vi "Part 1.vi"(11 "Input":string) -> (3 "Output":i64)   [LabVIEW 2021]
uses:
  d659a181-ebe8-414d-ab0f-685b255bff87.vi
  4776c344-dbbc-458a-98bd-0c10030d5930.vi
  <userlib>/_OpenG.lib/string/string.llb/Convert EOLs (String)__ogtk.vi
  <vilib>/Comparison/Less/Less Functor/Less Functor.lvclass
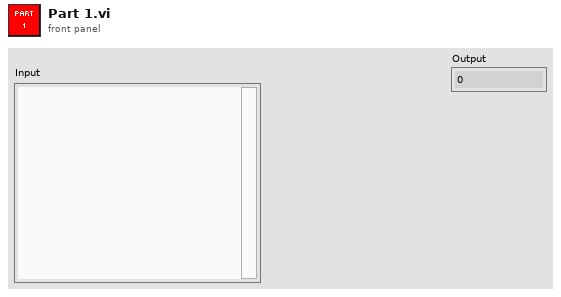
[diagram p1: front panel]
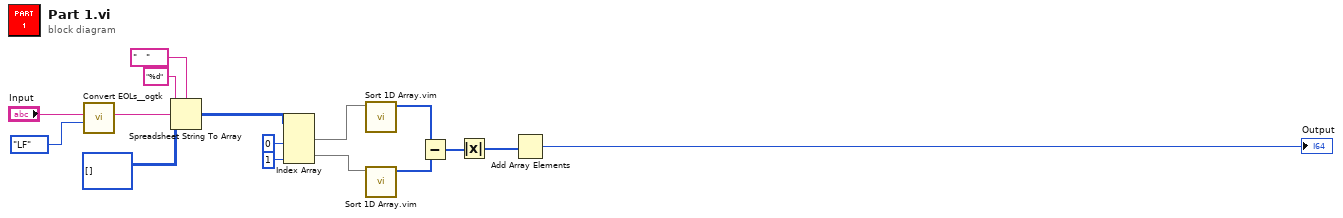
[diagram p0: block diagram]
diagram:
  n1 = call-poly <userlib>:"Convert EOLs__ogtk.vi"("Convert to:"=enum16{"CR", "LF", "CRLF"}."LF", "String in"="Input") -> ("String out"=w12:string)  [unwired: 9 in]
  n2 = Spreadsheet String To Array(delimiter (Tab)="   ", format string="%d", spreadsheet string=w12, array type (2D Dbl)=i64[][] []) -> (array=w10:i64[][])
  n3 = Index Array(array=w10, index (col) #1=0 ("disabled index (col)"), index (col) #2=1 ("index (col)")) -> (element #1=w7:i64[], element #2=w6:i64[])  [unwired: 2 in]
  n4 = call "Sort 1D Array.vim"("unsorted array"=w7) -> ("sorted array"=w5:i64[])  [unwired: 10 in]
  n5 = call "Sort 1D Array.vim"("unsorted array"=w6) -> ("sorted array"=w4:i64[])  [unwired: 10 in]
  n6 = Subtract(x=w5, y=w4) -> (x-y=w3:i64[])
  n7 = Absolute Value(x=w3) -> (abs(x)=w2:i64[])
  n8 = Add Array Elements(numeric array=w2) -> (sum=→"Output":i64)
